vi "Shooter-firstVI.vi"(0 "bottomWheelMotor":T4={"DeviceStatus"={"status"=FALSE, "code"=0, "source"=""}, "Type"=enum."PWM", "PWM"={"PWM Channel"=enum."Invalid", "DeadBand"={"Name"="", "maxPositivePwm"=0, "minPositivePwm"=0, "centerPwm"=0, "maxNegativePwm"=0, "minNegativePwm"=0, "angularRange"=0}}, "CAN"={"Device Number"=0, "SetOutput VI Ref"=variant(enum8{"Percent VBus", "Current", "Speed", "Position", "Voltage"} enum."Percent VBus"), "GetOutput VI Ref"=variant(refnum<k1> refnum), "Enable VI Ref"=variant(dbl 12.0), "Disable VI Ref"=variant(enum8{"Percent VBus", "Speed", "Position", "Slave", "Unchanged / Invalid"} enum."Percent VBus"), "Data"=variant}, "Invert"=FALSE}, 1 "RpmStableVal":dbl, 2 "RpmThreshold":dbl, 3 "topInvert":bool, 5 "topWheelMotor":T4={"DeviceStatus"={"status"=FALSE, "code"=0, "source"=""}, "Type"=enum."PWM", "PWM"={"PWM Channel"=enum."Invalid", "DeadBand"={"Name"="", "maxPositivePwm"=0, "minPositivePwm"=0, "centerPwm"=0, "maxNegativePwm"=0, "minNegativePwm"=0, "angularRange"=0}}, "CAN"={"Device Number"=0, "SetOutput VI Ref"=variant(enum8{"Percent VBus", "Current", "Speed", "Position", "Voltage"} enum."Percent VBus"), "GetOutput VI Ref"=variant(refnum<k1> refnum), "Enable VI Ref"=variant(dbl 12.0), "Disable VI Ref"=variant(enum8{"Percent VBus", "Speed", "Position", "Slave", "Unchanged / Invalid"} enum."Percent VBus"), "Data"=variant}, "Invert"=FALSE}, 9 "topWheel":T3, 11 "bottomWheel":T8, 12 "topPIDF":T2, 13 "bottomPIDF":T1, 14 "bottomInvert":bool) -> (4 "done":bool)   [LabVIEW 2016]
uses:
  <vilib>/Rock Robotics/WPI/MotorControl/WPI_MotorControlDeviceRef.ctl
  <vilib>/Rock Robotics/WPI/MotorControl/WPI_MotorControlType.ctl
  <vilib>/Rock Robotics/SystemInterfaces/DIO/FPGA_DIOPWMChannel.ctl
  <vilib>/Rock Robotics/WPI/PWM/WPI_PWMDeadband.ctl
  <vilib>/Rock Robotics/WPI/ThirdParty/CanMotor/TalonSRX/WPI_CANTalonSRX_APIControlMode.ctl
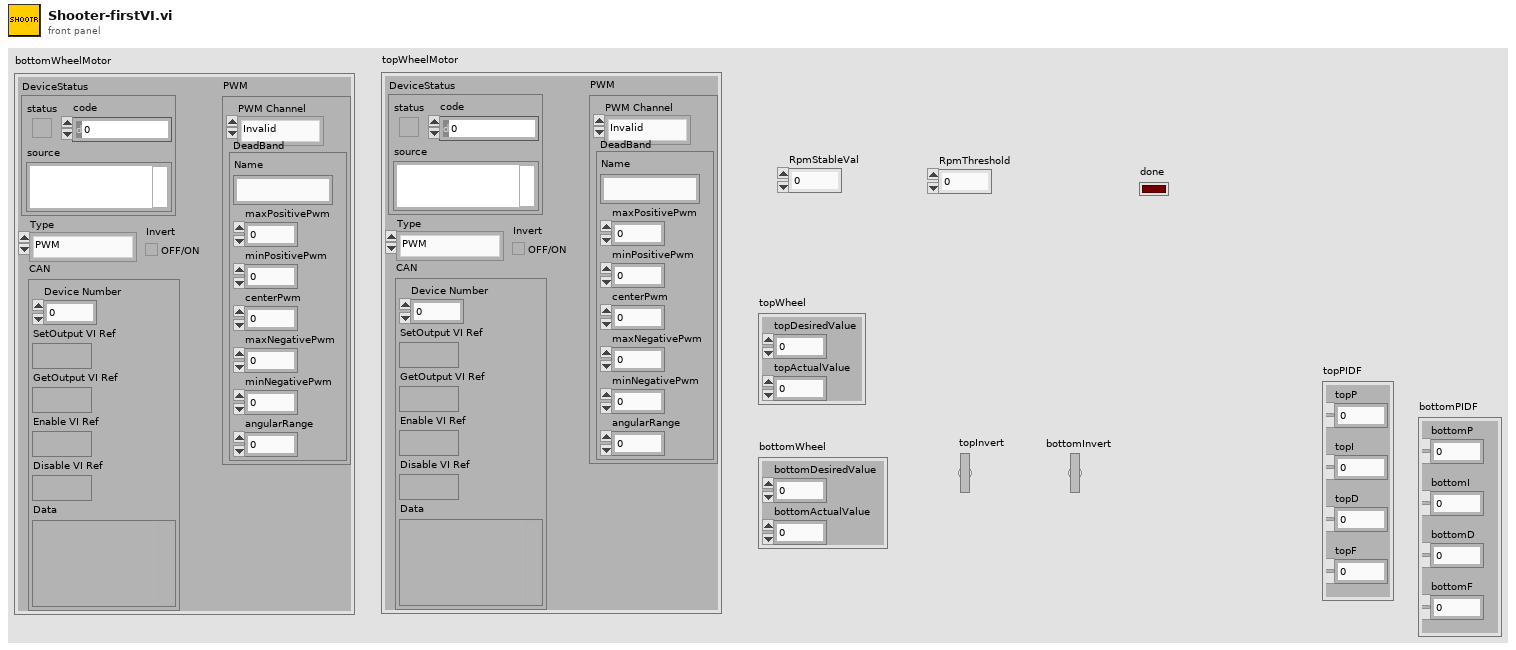
[diagram p1: front panel]
types:
  T1 = cluster{"bottomP":dbl, "bottomI":dbl, "bottomD":dbl, "bottomF":dbl}
  T2 = cluster{"topP":dbl, "topI":dbl, "topD":dbl, "topF":dbl}
  T3 = cluster{"topDesiredValue":dbl, "topActualValue":dbl}
  T4 = typedef "WPI_MotorControlDeviceRef.ctl" = cluster{"DeviceStatus":errorcluster, "Type":T5, "PWM":cluster{"PWM Channel":T6, "DeadBand":T7}, "CAN":cluster{"Device Number":u8, "SetOutput VI Ref":variant, "GetOutput VI Ref":variant, "Enable VI Ref":variant, "Disable VI Ref":variant, "Data":variant}, "Invert":bool}
  T5 = typedef "WPI_MotorControlType.ctl" = enum16{"PWM", "CAN"}
  T6 = typedef "FPGA_DIOPWMChannel.ctl" = enum8{"PWM 0", "PWM 1", "PWM 2", "PWM 3", "PWM 4", "PWM 5", "PWM 6", "PWM 7", "PWM 8", "PWM 9", "PWM MXP 0", "PWM MXP 1", "PWM MXP 2", "PWM MXP 3", "PWM MXP 4", "PWM MXP 5", "PWM MXP 6", "PWM MXP 7", "PWM MXP 8", "PWM MXP 9", "Invalid"}
  T7 = typedef "WPI_PWMDeadband.ctl" = cluster{"Name":string, "maxPositivePwm":i32, "minPositivePwm":i32, "centerPwm":i32, "maxNegativePwm":i32, "minNegativePwm":i32, "angularRange":u16}
  T8 = cluster{"bottomDesiredValue":dbl, "bottomActualValue":dbl}
  T9 = typedef "WPI_CANTalonSRX_APIControlMode.ctl" = enum8{"Percent VBus", "Speed", "Position", "Slave", "Unchanged / Invalid", "Voltage Compensation", "Current", "Motion Profile", "Motion Magic"}
  T10 = cluster{"bottomP":bool, "bottomI":bool, "bottomD":bool, "bottomF":bool}
  T11 = cluster{"topP":bool, "topI":bool, "topD":bool, "topF":bool}
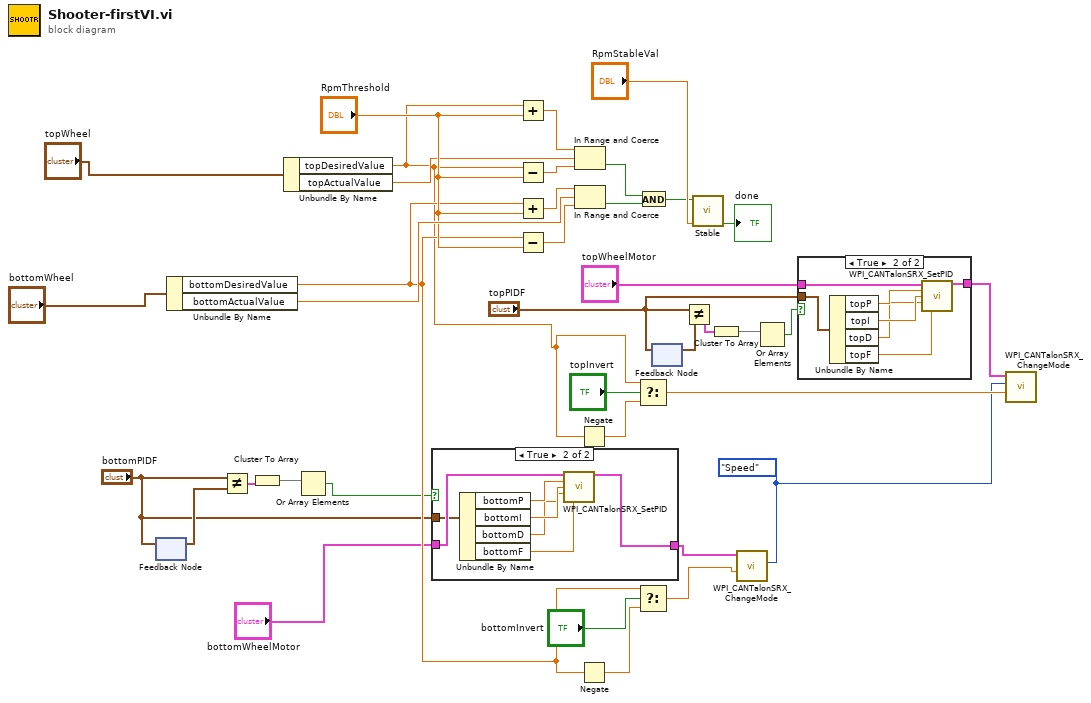
[diagram p0: block diagram]
diagram:
  w8 = WPI_CANTalonSRX_APIControlMode."Speed" ("Control Mode")
  n1 = feedback-in #1("bottomPIDF") -> ()
  n2 = feedback #1() -> (w15:T1)  [unwired: 1 in]
  n3 = Unbundle By Name("bottomWheel") -> ("bottomDesiredValue"=w19:dbl, "bottomActualValue"=w30:dbl)
  n4 = Not Equal?(x="bottomPIDF", y=w15) -> (x != y?=w14:T10)
  n5 = Cluster To Array(cluster=w14) -> (array=w13:bool[])
  n6 = Unbundle By Name("topWheel") -> ("topDesiredValue"=w10:dbl, "topActualValue"=w24:dbl)
  n7 = Or Array Elements(Boolean array=w13) -> (logical OR=w12:bool)
  n8 = case shown="True" w12 {
    tunnel: "bottomWheelMotor" -> [w38 w45]
    tunnel: [w38 w44] -> w17
    tunnel: "bottomPIDF" -> [_ w43]
    frame False {
    }
    frame True {
      n9 = Unbundle By Name(w43) -> ("bottomP"=w42:dbl, "bottomI"=w41:dbl, "bottomD"=w40:dbl, "bottomF"=w39:dbl)
      n10 = call <vilib>:"WPI_CANTalonSRX_SetPID.vi"("CAN Talon SRX Ref"=w45, "P"=w42, "I"=w41, "D"=w40, "F"=w39) -> ("CAN Talon SRX Ref"=w44:T4)  [unwired: 9 in, 1 out]
    }
  }
  n11 = Add(x=w10, y="RpmThreshold") -> (x+y=w26:dbl)
  n12 = Subtract(x=w10, y="RpmThreshold") -> (x-y=w27:dbl)
  n13 = Add(x=w19, y="RpmThreshold") -> (x+y=w32:dbl)
  n14 = Subtract(x=w19, y="RpmThreshold") -> (x-y=w31:dbl)
  n15 = In Range and Coerce(upper limit=w26, x=w24, lower limit=w27) -> (In Range?=w28:bool)  [unwired: 1 out]
  n16 = In Range and Coerce(upper limit=w32, x=w30, lower limit=w31) -> (In Range?=w29:bool)  [unwired: 1 out]
  n17 = Negate(x=w10) -> (-x=w36:dbl)
  n18 = Negate(x=w19) -> (-x=w34:dbl)
  n19 = Select(t=w10, s="topInvert", f=w36) -> (s? t:f=w16:dbl)
  n20 = Select(t=w19, s="bottomInvert", f=w34) -> (s? t:f=w20:dbl)
  n21 = And(x=w28, y=w29) -> (x .and. y?=w21:bool)
  n22 = feedback #2() -> (w6:T2)  [unwired: 1 in]
  n23 = feedback-in #2("topPIDF") -> ()
  n24 = Not Equal?(x="topPIDF", y=w6) -> (x != y?=w4:T11)
  n25 = call <userlib>:"Stable.vi"("Eval Period (sec)"="RpmStableVal", "Signal Input"=w21) -> ("Stable"=→"done":bool)  [unwired: 9 in]
  n26 = Cluster To Array(cluster=w4) -> (array=w5:bool[])
  n27 = call <vilib>:"WPI_CANTalonSRX_ChangeMode.vi"("Output"=w20, "Control Mode"=w8, "CAN Talon SRX Ref"=w17) -> ()  [unwired: 7 in, 2 out]
  n28 = Or Array Elements(Boolean array=w5) -> (logical OR=w2:bool)
  n29 = case shown="True" w2 {
    tunnel: "topWheelMotor" -> [w46 w53]
    tunnel: [w46 w52] -> w3
    tunnel: "topPIDF" -> [_ w51]
    frame False {
    }
    frame True {
      n30 = Unbundle By Name(w51) -> ("topP"=w50:dbl, "topI"=w49:dbl, "topD"=w48:dbl, "topF"=w47:dbl)
      n31 = call <vilib>:"WPI_CANTalonSRX_SetPID.vi"("CAN Talon SRX Ref"=w53, "P"=w50, "I"=w49, "D"=w48, "F"=w47) -> ("CAN Talon SRX Ref"=w52:T4)  [unwired: 9 in, 1 out]
    }
  }
  n32 = call <vilib>:"WPI_CANTalonSRX_ChangeMode.vi"("Output"=w16, "Control Mode"=w8, "CAN Talon SRX Ref"=w3) -> ()  [unwired: 7 in, 2 out]
